vi "Launch Views.vi"(8 "error in (no error)":errorcluster, 10 "Full Factory in":refnum<class "Full Factory.lvclass">, 11 "UI Controller in":refnum<class "UI Controller.lvclass">) -> (0 "error out":errorcluster, 3 "UI Controller out":refnum<class "UI Controller.lvclass">)   [LabVIEW 2020, in "UI Controller.lvlib" / "Full Factory.lvclass"]
uses:
  Full Factory.lvclass
  UI Controller/UI Controller.lvclass
panel:
  # "NOTICE -- YOU MUST LEAVE THIS NOTICE IN PLACE.\n\nCopyright (c) 2017, LIANG LIU Shawn.Liu.cn@gmail.com\nAll rights reserved.\n\nRedistribution and use in source and binary forms, with or without modification, are permitted provided that the following conditions are met:\n-Redistributions of source code must retain the above copyright notice, this list of conditions and the following disclaimer.\n-Redistributions in binary form must reproduce the above copyright notice, this list of conditions and the following disclaimer in the documentation and/or other materials provided with the distribution.\n-Neither the name of the eLp nor the names of its contributors may be used to endorse or promote products derived from this software without specific prior written permission.\n\nTHIS SOFTWARE IS PROVIDED BY THE COPYRIGHT HOLDERS AND CONTRIBUTORS \"AS IS\" AND ANY EXPRESS OR IMPLIED WARRANTIES, INCLUDING, BUT NOT LIMITED TO, THE IMPLIED WARRANTIES OF MERCHANTABILITY AND FITNESS FOR A PARTICULAR PURPOSE ARE DISCLAIMED. IN NO EVENT SHALL THE COPYRIGHT HOLDER OR CONTRIBUTORS BE LIABLE FOR ANY DIRECT, INDIRECT, INCIDENTAL, SPECIAL, EXEMPLARY, OR CONSEQUENTIAL DAMAGES (INCLUDING, BUT NOT LIMITED TO, PROCUREMENT OF SUBSTITUTE GOODS OR SERVICES; LOSS OF USE, DATA, OR PROFITS; OR BUSINESS INTERRUPTION) HOWEVER CAUSED AND ON ANY THEORY OF LIABILITY, WHETHER IN CONTRACT, STRICT LIABILITY, OR TORT (INCLUDING NEGLIGENCE OR OTHERWISE) ARISING IN ANY WAY OUT OF THE USE OF THIS SOFTWARE, EVEN IF ADVISED OF THE POSSIBILITY OF SUCH DAMAGE."
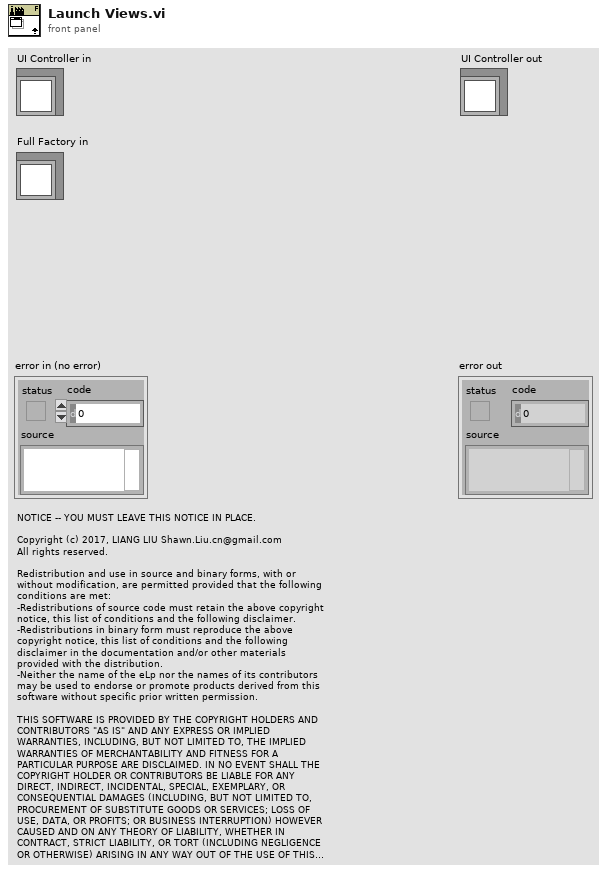
[diagram p1: front panel]
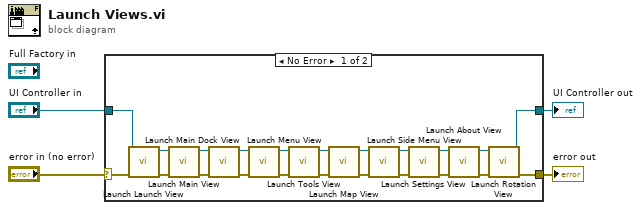
[diagram p0: block diagram]
diagram:
  n1 = case shown="No Error" "error in (no error)" {
    selector: "error in (no error)" -> [w26 w28]
    tunnel: "UI Controller in" -> [w25 w27]
    tunnel: [w7 w28] -> w2
    tunnel: [w5 w27] -> w1
    frame No Error {
      n2 = call "Launch Launch View.vi"("error in (no error)"=w26, "UI Controller in"=w25) -> ("error out"=w22:errorcluster, "UI Controller out"=w23:refnum<class "UI Controller.lvclass">)  [unwired: 8 in]
      n3 = call "Launch Main View.vi"("error in (no error)"=w22, "UI Controller in"=w23) -> ("error out"=w20:errorcluster, "UI Controller out"=w21:refnum<class "UI Controller.lvclass">)  [unwired: 8 in]
      n4 = call "Launch Main Dock View.vi"("error in (no error)"=w20, "UI Controller in"=w21) -> ("error out"=w18:errorcluster, "UI Controller out"=w19:refnum<class "UI Controller.lvclass">)  [unwired: 8 in]
      n5 = call "Launch Menu View.vi"("error in (no error)"=w18, "UI Controller in"=w19) -> ("error out"=w16:errorcluster, "UI Controller out"=w17:refnum<class "UI Controller.lvclass">)  [unwired: 8 in]
      n6 = call "Launch Tools View.vi"("error in (no error)"=w16, "UI Controller in"=w17) -> ("error out"=w14:errorcluster, "UI Controller out"=w15:refnum<class "UI Controller.lvclass">)  [unwired: 8 in]
      n7 = call "Launch Map View.vi"("error in (no error)"=w14, "UI Controller in"=w15) -> ("error out"=w12:errorcluster, "UI Controller out"=w13:refnum<class "UI Controller.lvclass">)  [unwired: 8 in]
      n8 = call "Launch Side Menu View.vi"("error in (no error)"=w12, "UI Controller in"=w13) -> ("error out"=w10:errorcluster, "UI Controller out"=w11:refnum<class "UI Controller.lvclass">)  [unwired: 8 in]
      n9 = call "Launch Settings View.vi"("error in (no error)"=w10, "UI Controller in"=w11) -> ("error out"=w8:errorcluster, "UI Controller out"=w9:refnum<class "UI Controller.lvclass">)  [unwired: 8 in]
      n10 = call "Launch About View.vi"("error in (no error)"=w8, "UI Controller in"=w9) -> ("error out"=w24:errorcluster, "UI Controller out"=w6:refnum<class "UI Controller.lvclass">)  [unwired: 8 in]
      n11 = call "Launch Rotation View.vi"("error in (no error)"=w24, "UI Controller in"=w6) -> ("error out"=w7:errorcluster, "UI Controller out"=w5:refnum<class "UI Controller.lvclass">)  [unwired: 8 in]
    }
    frame Error {
    }
  }
  "error out" <- w2
  "UI Controller out" <- w1
